vi "Main.vi"() -> ()   [LabVIEW 2023, in "SwitchExecController.lvlib"]
uses:
  SwitchExecController.lvlib
  PluginSDK/Plugin Session.lvclass
  PluginSDK/Plugin Events Enum.ctl
  PluginSDK/InstrumentStudio Plugin SDK.lvlib
panel:
  in  "Session Id":u64
  in  "Routes":i32[](listbox)
  in  "Multiconnect Mode:":i32(ring) items=["No Multiconnect"=0, "Multiconnect Routes"=1, "Use Default Setting for Route"=-1]
  in  "Operation:":T1(ring)
  in  "Switch Executive Virtual Device:":string(combo)
  out "Status":string
  in  "Run":bool
  # "SWITCH EXECUTIVE"
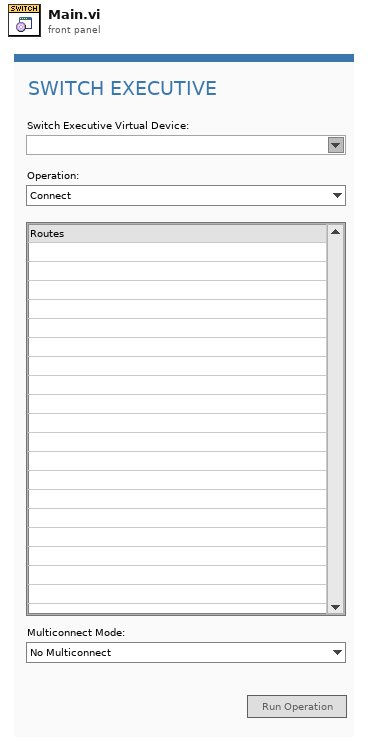
[diagram p1: front panel]
types:
  T1 = enum16{"Connect", "Disconnect", "Disconnect All"}
  T2 = enum8{"Enabled", "Disabled", "Disabled and Grayed Out"}
  T3 = enum16{"Connect", "Disconnect", "Disconnect All", "Connect & Disconnect"}
  T4 = typedef "InstrumentStudio Plugin SDK.lvlib/Plugin Events Enum.ctl" = enum16{"Shutdown", "Project Saved", "Stop All Outputs"}
  T5 = typedef "InstrumentStudio Plugin SDK.lvlib/Event Registration Refnum.ctl" = refnum<event-registration>
  T6 = typedef "niSE SessionRefnum.ctl" = refnum<k1>
  T7 = cluster{"Multiconnect Mode: ":refnum<vi>, "Disabled":enum8{"Enabled", "Disabled", "Disabled and Grayed Out"}}
  T8 = cluster{"Routes":refnum<vi>, "Disabled":enum8{"Enabled", "Disabled", "Disabled and Grayed Out"}}
  T9 = cluster{"Multiconnect Mode: ":refnum<vi>, "Disabled":enum8{"Enabled", "Disabled", "Disabled and Grayed Out"}}[]
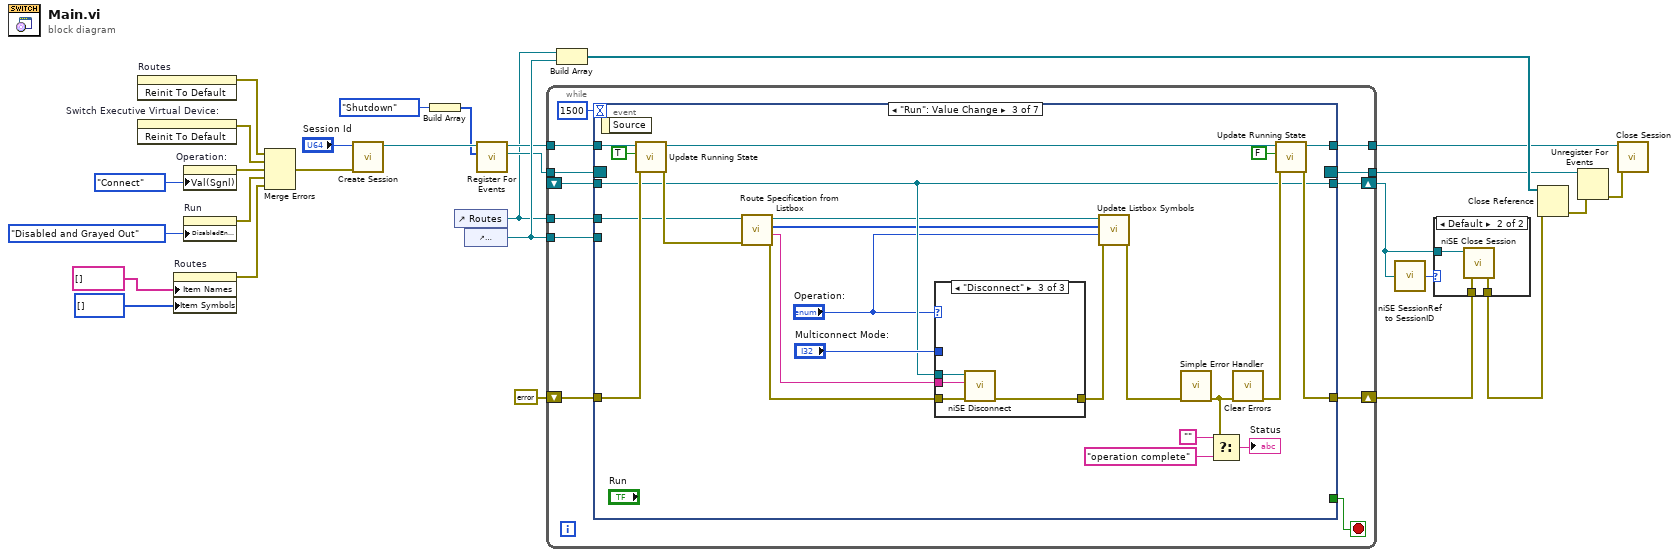
[diagram p0: block diagram]
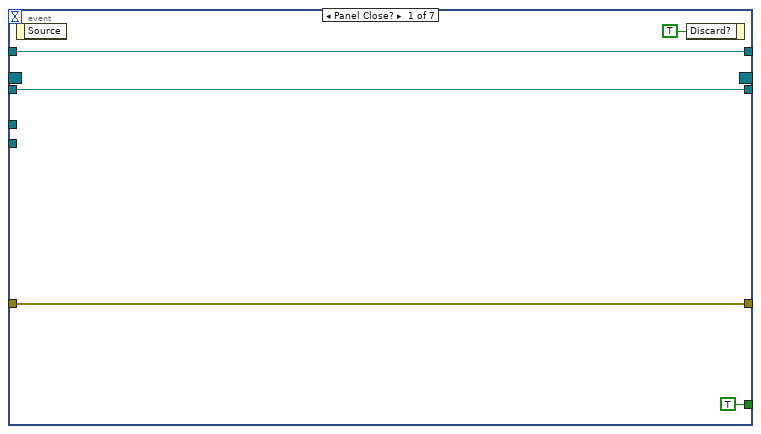
[diagram p2: hidden frame]
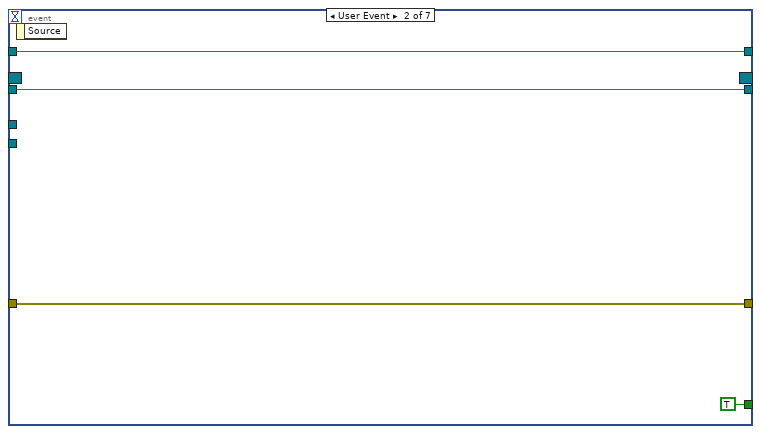
[diagram p3: hidden frame]
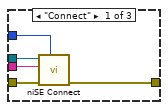
[diagram p4: hidden frame]
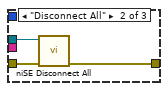
[diagram p5: hidden frame]
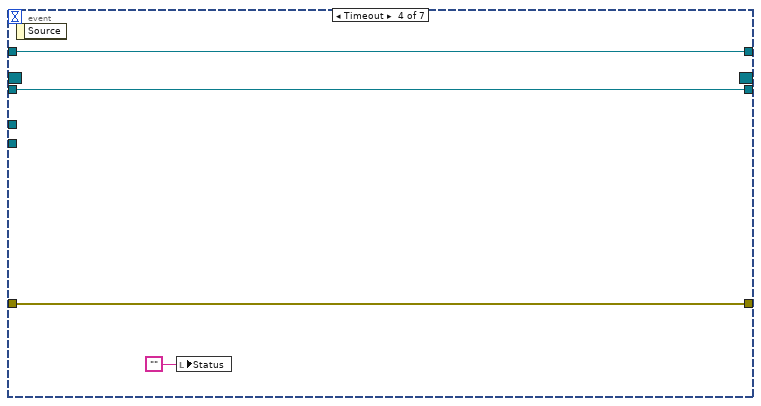
[diagram p6: hidden frame]
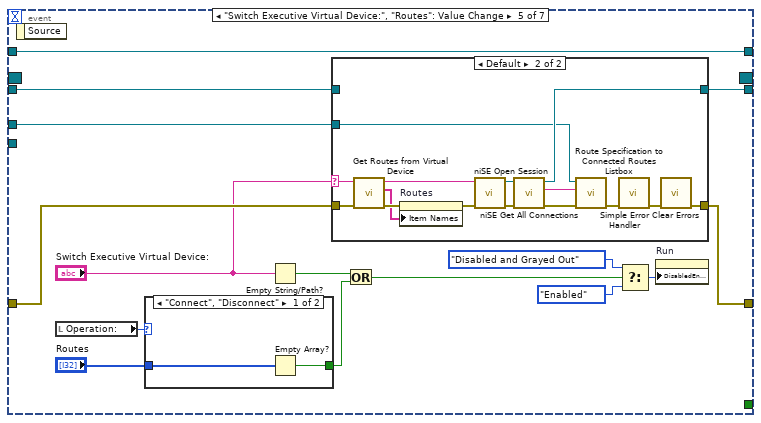
[diagram p7: hidden frame]
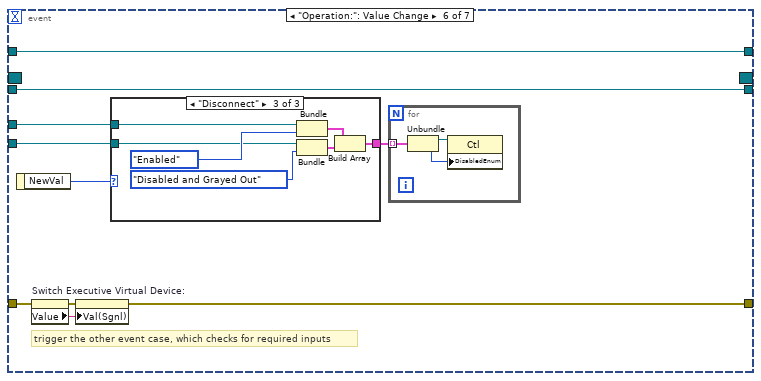
[diagram p10: hidden frame]
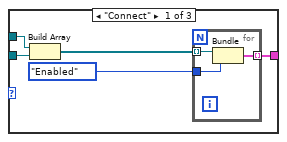
[diagram p11: hidden frame]
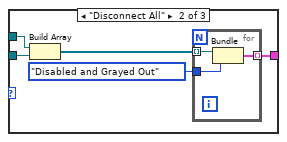
[diagram p12: hidden frame]
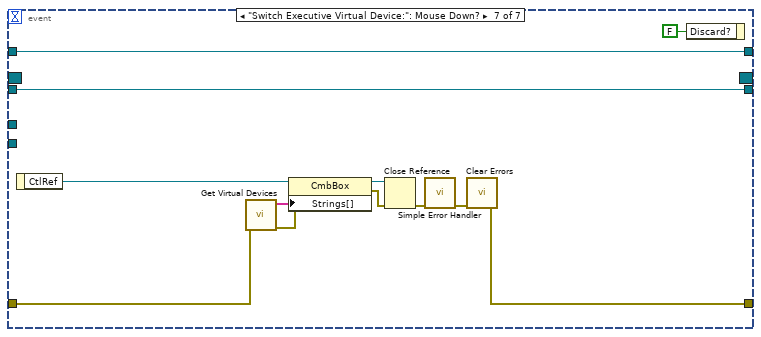
[diagram p13: hidden frame]
diagram:
  n1 = invoke on="Routes" class="LstBox (strict)" method="Reinit To Default"() -> (error out=w2:errorcluster)  [unwired: 3 in, 2 out]
  n2 = invoke on="Switch Executive Virtual Device:" class="CmbBox" method="Reinit To Default"() -> (error out=w4:errorcluster)  [unwired: 3 in, 2 out]
  n3 = property on="Routes" class="LstBox (strict)"("Item Names"=string[] [], "Item Symbols"=i32[] []) -> (error out=w1:errorcluster)  [unwired: 2 in, 1 out]
  n4 = property on="Operation:" class="Enum (strict)"("Val(Sgnl)"=T3."Connect" ("Value (Signaling)")) -> (error out=w5:errorcluster)  [unwired: 2 in, 1 out]
  n5 = property on="Run" class="Bool"("DisabledEnum"=T2."Disabled and Grayed Out" ("Disabled")) -> (error out=w3:errorcluster)  [unwired: 2 in, 1 out]
  n6 = Merge Errors(w2, w4, w5, w3, w1) -> (w10:errorcluster)
  n7 = call "Create Session.vi"("error in (no error)"=w10, "Session Id"="Session Id") -> ("Session out"=w27:refnum<class "Plugin Session.lvclass">)  [unwired: 5 in, 4 out]
  n8 = Build Array(Plugin_Events_Enum."Shutdown" ("Events")) -> (w25:T4[])
  n9 = control-ref of="Routes"() -> (w16:refnum<vi>)
  n10 = control-ref of="Multiconnect Mode:"() -> (w23:refnum<vi>)
  n11 = call "Register For Events.vi"("Events To Register"=w25, "Session in"=w27) -> ("Event Refnum"=w21:T5, "Session out"=w22:refnum<class "Plugin Session.lvclass">)  [unwired: 7 in, 1 out]
  n12 = while {
    tunnel: w22 -> [w40]
    tunnel: [w39] -> w18
    tunnel: w21 -> [w38]
    tunnel: w16 -> [w36]
    tunnel: w23 -> [w35]
    tunnel: [w34] -> w17
    shift-right: [w33] -> w15
    shift-left: errorcluster {"status"=FALSE, "code"=0, "source"=""} ("error out") -> [w32]
    shift-right: [w30] -> w12
    shift-left: _ -> [w31]
    stop <- w37 stop-if-true
    n13 = event shown="[2] \"Run\": Value Change" {
      selector: w38 -> [_ _ _ _ _ _ _]
      dyn-events: [_ _ _ _ _ _ _] -> w34
      timeout: 1500 -> [_ _ _ _ _ _ _]
      tunnel: w40 -> [w44 w49 w72 w88 w103 w133 w171]
      tunnel: [w44 w49 w69 w88 w103 w133 w171] -> w39
      tunnel: [TRUE TRUE _ _ _ _ _] -> w37
      tunnel: w36 -> [_ _ w62 _ w90 w126 _]
      tunnel: w35 -> [_ _ _ _ _ w125 _]
      tunnel: [w43 w48 w65 w85 w94 w129 w162] -> w33
      tunnel: w32 -> [w43 w48 w64 w85 w95 w131 w161]
      tunnel: w31 -> [w42 w47 w61 w86 w89 w128 w160]
      tunnel: [w42 w47 w61 w86 w93 w128 w160] -> w30
      event Panel Close? {
        n14 = event-data() -> ()  [unwired: 1 in, 1 out]
        n15 = event-data("Discard?"=TRUE) -> ()  [unwired: 1 in, 1 out]
      }
      event User Event {
        n16 = event-data() -> ()  [unwired: 1 in, 1 out]
      }
      event "Run": Value Change {
        n17 = event-data() -> ()  [unwired: 1 in, 1 out]
        n18 = call "Update Running State.vi"("error in (no error)"=w64, "Is Running"=TRUE, "Plugin Session in"=w72) -> ("error out"=w63:errorcluster, "Plugin Session out"=w68:refnum<class "Plugin Session.lvclass">)  [unwired: 7 in]
        n19 = call "Route Specification from Listbox.vi"("error in (no error)"=w63, "listbox reference"=w62) -> ("error out"=w52:errorcluster, "route specification"=w53:string, "Indices of Routes"=w51:i32[], "listbox reference out"=w56:refnum<vi>)  [unwired: 6 in]
        n20 = case shown="\"Disconnect\"" "Operation:" {
          tunnel: w61 -> [w77 w80 w84]
          tunnel: w52 -> [w76 w79 w83]
          tunnel: "Multiconnect Mode:" -> [w75 _ _]
          tunnel: [w73 w78 w81] -> w54
          tunnel: w53 -> [w74 _ w82]
          frame "Connect" {
            n21 = call <vilib>:"niSE Connect.vi"("Multiconnect Mode (Use Default Mode)"=w75, "error in (no error)"=w76, "Connection Specification (\"\")"=w74, "NISE Session (in)"=w77) -> ("error out"=w73:errorcluster)  [unwired: 6 in, 1 out]
          }
          frame "Disconnect All" {
            n22 = call <vilib>:"niSE Disconnect All.vi"("error in (no error)"=w79, "NISE Session (in)"=w80) -> ("error out"=w78:errorcluster)  [unwired: 4 in, 1 out]
          }
          frame "Disconnect" {
            n23 = call <vilib>:"niSE Disconnect.vi"("error in (no error)"=w83, "Disconnection Specification (\"\")"=w82, "NISE Session (in)"=w84) -> ("error out"=w81:errorcluster)  [unwired: 3 in, 1 out]
          }
        }
        n24 = call "Update Listbox Symbols.vi"("error in (no error)"=w54, "Operation"="Operation:", "Indices to change"=w51, "ListBox in"=w56) -> ("error out"=w55:errorcluster)  [unwired: 6 in, 1 out]
        n25 = call <vilib>:"Simple Error Handler.vi"("error in (no error)"=w55) -> ("error out"=w60:errorcluster)  [unwired: 4 in, 4 out]
        n26 = Select(t="", s=w60, f="operation complete" ("String")) -> (s? t:f=→"Status":string)
        n27 = call <vilib>:"Clear Errors.vi"("error in (no error)"=w60) -> ("error out"=w66:errorcluster)  [unwired: 5 in, 1 out]
        n28 = call "Update Running State.vi"("error in (no error)"=w66, "Is Running"=FALSE, "Plugin Session in"=w68) -> ("error out"=w65:errorcluster, "Plugin Session out"=w69:refnum<class "Plugin Session.lvclass">)  [unwired: 7 in]
      }
      event Timeout {
        n29 = event-data() -> ()  [unwired: 1 in, 1 out]
        n30 = local write "Status"("") -> ()
      }
      event "Switch Executive Virtual Device:", "Routes": Value Change {
        n31 = event-data() -> ()  [unwired: 1 in, 1 out]
        n32 = local read "Operation:"() -> (w102:T1)
        n33 = case shown="\"Connect\", \"Disconnect\"" w102 {
          tunnel: "Routes" -> [w122 _]
          tunnel: [w121 FALSE] -> w100
          frame "Connect", "Disconnect" {
            n34 = Empty Array?(array=w122) -> (empty?=w121:bool)
          }
          frame "Disconnect All" {
          }
        }
        n35 = Empty String/Path?(string/path="Switch Executive Virtual Device:") -> (empty?=w101:bool)
        n36 = case shown="Default" "Switch Executive Virtual Device:" {
          selector: "Switch Executive Virtual Device:" -> [_ w115]
          tunnel: w95 -> [w105 w119]
          tunnel: [w105 w118] -> w94
          tunnel: w89 -> [w104 _]
          tunnel: [w104 w111] -> w93
          tunnel: w90 -> [_ w108]
          frame "" {
          }
          frame Default {
            n37 = call "Get Routes from Virtual Device.vi"("error in"=w119, "Virtual Device"=w115) -> ("error out"=w117:errorcluster, "Routes"=w116:string[], "Virtual Device out"=w114:string)  [unwired: 6 in]
            n38 = property on="Routes" class="LstBox (strict)"(error in=w117, "Item Names"=w116) -> (error out=w106:errorcluster)  [unwired: 1 in, 1 out]
            n39 = call <vilib>:"niSE Open Session.vi"("error in (no error)"=w106, "Virtual Device Name (SwitchConfiguration1)"=w114) -> ("error out"=w112:errorcluster, "NISE Session (out)"=w113:T6)  [unwired: 4 in]
            n40 = call <vilib>:"niSE Get All Connections.vi"("error in (no error)"=w112, "NISE Session (in)"=w113) -> ("error out"=w110:errorcluster, "Route Specification"=w107:string, "NISE Session (out)"=w111:T6)  [unwired: 3 in]
            n41 = call "Route Specification to Connected Routes Listbox.vi"("error in (no error)"=w110, "route specification"=w107, "listbox reference"=w108) -> ("error out"=w109:errorcluster)  [unwired: 7 in, 1 out]
            n42 = call <vilib>:"Simple Error Handler.vi"("error in (no error)"=w109) -> ("error out"=w120:errorcluster)  [unwired: 4 in, 4 out]
            n43 = call <vilib>:"Clear Errors.vi"("error in (no error)"=w120) -> ("error out"=w118:errorcluster)  [unwired: 5 in, 1 out]
          }
        }
        n44 = Or(x=w101, y=w100) -> (x .or. y?=w99:bool)
        n45 = Select(t=T2."Disabled and Grayed Out" ("Disabled"), s=w99, f=T2."Enabled" ("Disabled")) -> (s? t:f=w96:T2)
        n46 = property on="Run" class="Bool"("DisabledEnum"=w96) -> ()  [unwired: 2 in, 2 out]
      }
      event "Operation:": Value Change {
        # "trigger the other event case, which checks for required inputs"
        n47 = event-data() -> ("NewVal"=w127:T1)  [unwired: 1 in]
        n48 = property on="Switch Executive Virtual Device:" class="CmbBox"(error in=w131) -> (error out=w130:errorcluster, "Value"=w132:string)  [unwired: 1 in, 1 out]
        n49 = property on="Switch Executive Virtual Device:" class="CmbBox"(error in=w130, "Val(Sgnl)"=w132) -> (error out=w129:errorcluster)  [unwired: 1 in, 1 out]
        n50 = case shown="\"Disconnect\"" w127 {
          tunnel: w126 -> [w138 w146 w154]
          tunnel: w125 -> [w137 w145 w153]
          tunnel: [w134 w142 w152] -> w124
          frame "Connect" {
            n51 = Build Array(w138, w137) -> (w136:refnum<vi>[])
            n52 = for {
              tunnel: w136 -> [w141] mode=indexing
              tunnel: T2."Enabled" ("Disabled") -> [w140]
              tunnel: [w139] -> w134 mode=indexing
              n53 = Bundle("Multiconnect Mode:"=w141, "Disabled"=w140) -> (w139:T7)  [unwired: 1 in]
            }
          }
          frame "Disconnect All" {
            n54 = Build Array(w146, w145) -> (w144:refnum<vi>[])
            n55 = for {
              tunnel: w144 -> [w149] mode=indexing
              tunnel: T2."Disabled and Grayed Out" ("Disabled") -> [w148]
              tunnel: [w147] -> w142 mode=indexing
              n56 = Bundle("Multiconnect Mode:"=w149, "Disabled"=w148) -> (w147:T7)  [unwired: 1 in]
            }
          }
          frame "Disconnect" {
            n57 = Bundle("Routes"=w154, "Disabled"=T2."Enabled") -> (w151:T8)  [unwired: 1 in]
            n58 = Bundle("Multiconnect Mode:"=w153, "Disabled"=T2."Disabled and Grayed Out") -> (w150:T7)  [unwired: 1 in]
            n59 = Build Array(w151, w150) -> (w152:T9)
          }
        }
        n60 = for {
          tunnel: w124 -> [w159] mode=indexing
          n61 = Unbundle(w159) -> ("Multiconnect Mode:"=w158:refnum<vi>, "Disabled"=w157:T2)
          n62 = property on="Property Node" class="Ctl"(reference=w158, "DisabledEnum"=w157) -> ()  [unwired: 1 in, 2 out]
        }
      }
      event "Switch Executive Virtual Device:": Mouse Down? {
        n63 = event-data() -> ("CtlRef"=w169:refnum<vi>)  [unwired: 1 in]
        n64 = call "Get Virtual Devices.vi"("error in"=w161) -> ("error out"=w165:errorcluster, "Virtual Devices"=w166:string[])  [unwired: 9 in]
        n65 = property class="CmbBox"(reference=w169, error in=w165, "Strings[]"=w166) -> (reference out=w167:refnum<vi>, error out=w168:errorcluster)
        n66 = Close Reference(reference=w167, error in (no error)=w168) -> (error out=w164:errorcluster)
        n67 = call <vilib>:"Simple Error Handler.vi"("error in (no error)"=w164) -> ("error out"=w163:errorcluster)  [unwired: 4 in, 4 out]
        n68 = call <vilib>:"Clear Errors.vi"("error in (no error)"=w163) -> ("error out"=w162:errorcluster)  [unwired: 5 in, 1 out]
        n69 = event-data("Discard?"=FALSE) -> ()  [unwired: 1 in, 1 out]
      }
    }
  }
  n70 = Build Array(w16, w23) -> (w19:refnum<vi>[])
  n71 = call <vilib>:"niSE SessionRef to SessionID.vi"("NISE Session (in)"=w12) -> ("NISE Session ID"=w11:u32)  [unwired: 4 in]
  n72 = case shown="Default" w11 {
    tunnel: w12 -> [_ w175]
    tunnel: w15 -> [w172 w174]
    tunnel: [w172 w173] -> w14
    frame 0 {
    }
    frame Default {
      n73 = call <vilib>:"niSE Close Session.vi"("error in (no error)"=w174, "NISE Session (in)"=w175) -> ("error out"=w173:errorcluster)  [unwired: 5 in]
    }
  }
  n74 = Close Reference(reference=w19, error in (no error)=w14) -> (error out=w20:errorcluster)
  n75 = Unregister For Events(event registration refnum=w17, error in=w20) -> (error out=w24:errorcluster)
  n76 = call "Close Session.vi"("error in (no error)"=w24, "Session in"=w18) -> ()  [unwired: 9 in, 1 out]
